vi "Code1Ps.vi"(11 "Code1 In":string) -> (1 "紙箱號碼":string, 2 "機種代號":string, 3 "機種名":string)   [LabVIEW 2014]
panel:
  out "Array":string[](array[string])
  out "appended array":bool[](array[boolean])
  out "array":string[](array[string])
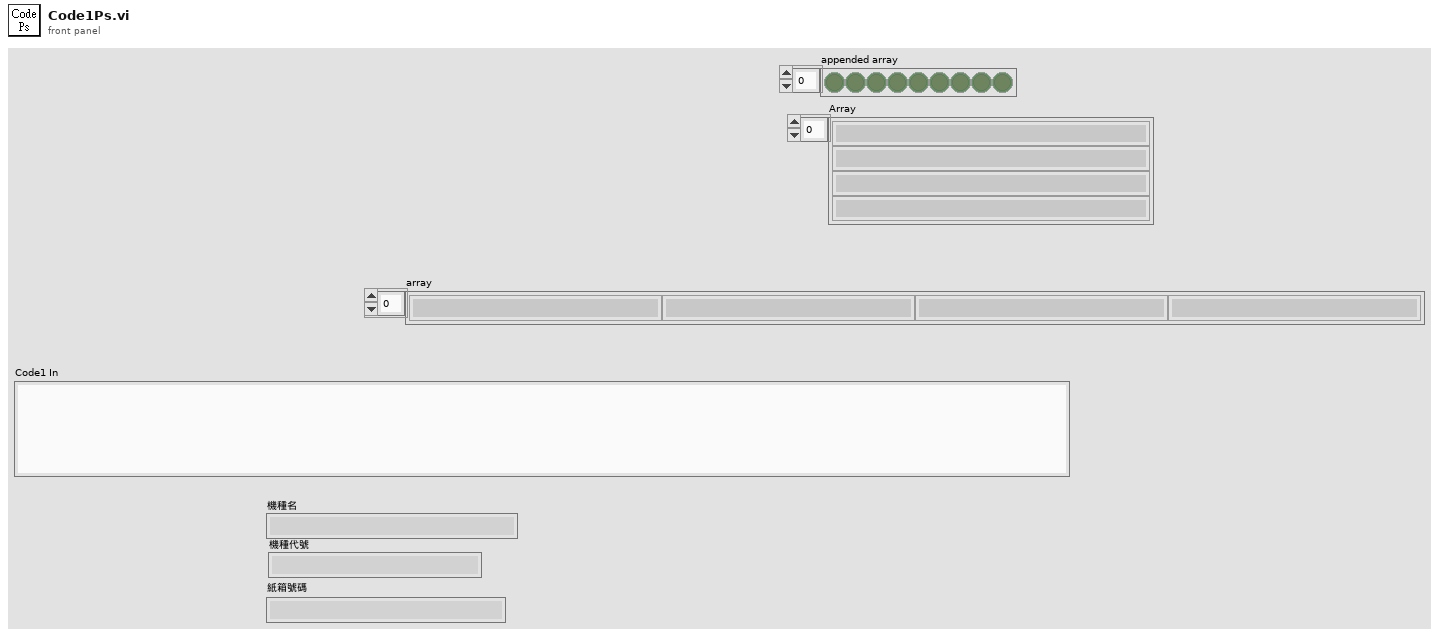
[diagram p1: front panel]
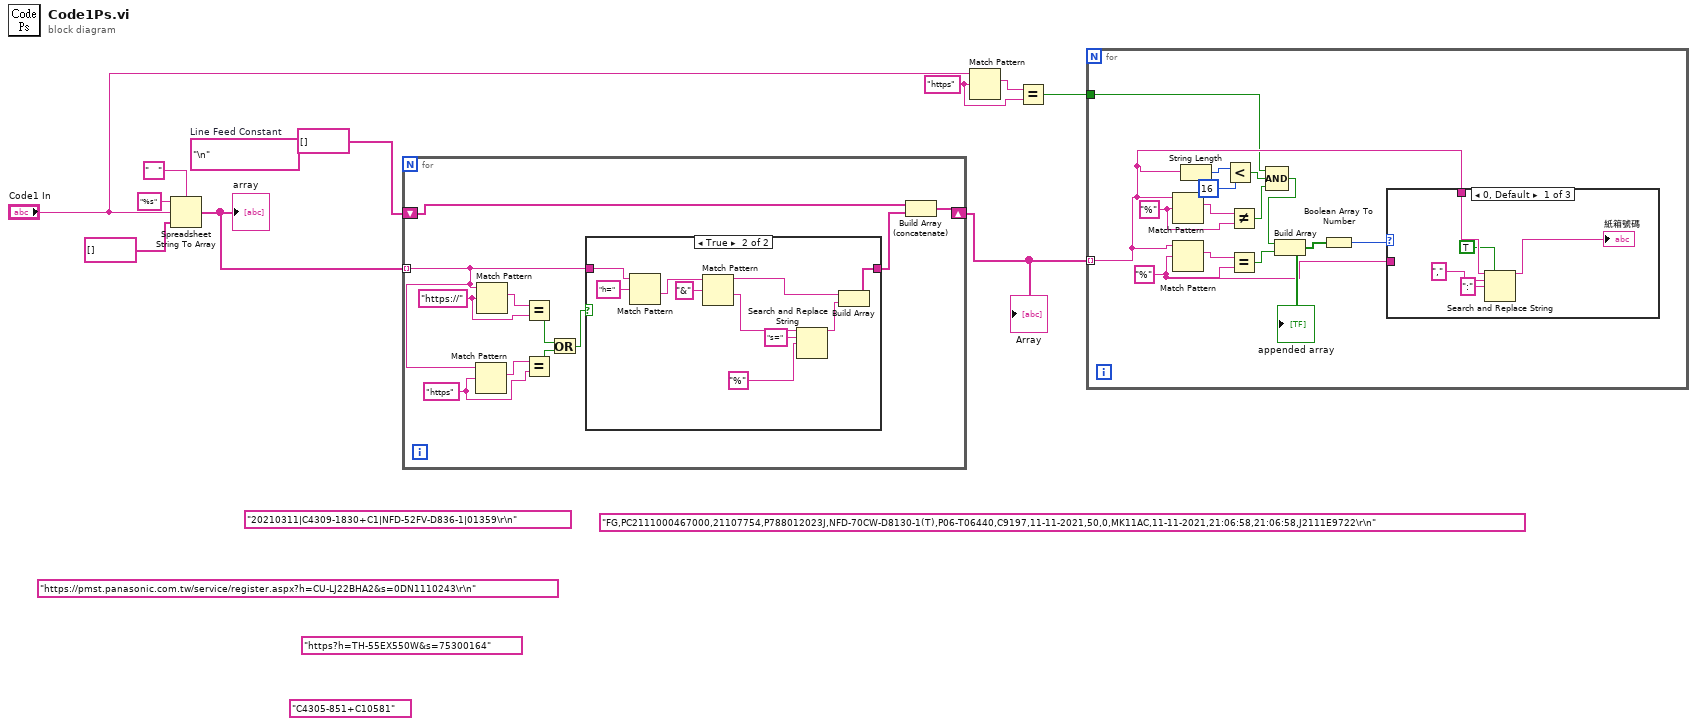
[diagram p0: block diagram]
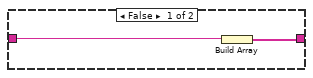
[diagram p2: hidden frame]
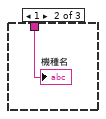
[diagram p3: hidden frame]
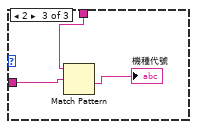
[diagram p4: hidden frame]
diagram:
  (unwired) "\n"  # Line Feed Constant
  (unwired) "FG,PC2111000467000,21107754,P788012023J,NFD-70CW-D8130-1(T),P06-T06440,C9197,11-11-2021,50,0,MK11AC,11-11-2021,21:06:58,21:06:58,J2111E9722\r\n" ("Code1 In")
  w3 = "https" ("regular expression")
  (unwired) "C4305-851+C10581"
  (unwired) "20210311|C4309-1830+C1|NFD-52FV-D836-1|01359\r\n" ("Code1 In")
  (unwired) "https://pmst.panasonic.com.tw/service/register.aspx?h=CU-LJ22BHA2&s=0DN1110243\r\n" ("Code1 In")
  (unwired) "https?h=TH-55EX550W&s=75300164" ("string")
  n1 = Spreadsheet String To Array(delimiter (Tab)="   ", format string="%s", spreadsheet string="Code1 In", array type (2D Dbl)=string[] []) -> (array=w8:string[])
  "array" <- w8
  n2 = for {
    tunnel: w8 -> [w16] mode=indexing
    shift-right: [w19] -> w6
    shift-left: string[] [] -> [w17]
    w14 = "https" ("regular expression")
    w21 = "https://" ("regular expression")
    n3 = Match Pattern(string=w16, regular expression=w14) -> (match substring=w15:string)  [unwired: 1 in, 3 out]
    n4 = Match Pattern(string=w16, regular expression=w21) -> (match substring=w20:string)  [unwired: 1 in, 3 out]
    n5 = Equal?(x=w20, y=w21) -> (x = y?=w13:bool)
    n6 = Equal?(x=w15, y=w14) -> (x = y?=w12:bool)
    n7 = Or(x=w13, y=w12) -> (x .or. y?=w11:bool)
    n8 = case shown="True" w11 {
      tunnel: [w22 w25] -> w18
      tunnel: w16 -> [w23 w24]
      frame False {
        n9 = Build Array(w23) -> (w22:string[])
      }
      frame True {
        n10 = Match Pattern(string=w24, regular expression="h=") -> (after substring=w27:string)  [unwired: 1 in, 3 out]
        n11 = Match Pattern(string=w27, regular expression="&") -> (before substring=w29:string, after substring=w30:string)  [unwired: 1 in, 2 out]
        n12 = Search and Replace String(input string=w30, search string="s=", replace string="%" ("replace string (\"\")")) -> (result string=w33:string)  [unwired: 5 in, 3 out]
        n13 = Build Array(w29, w33) -> (w25:string[])
      }
    }
    n14 = Build Array (concatenate)(w17, w18) -> (w19:string[])
  }
  "Array" <- w6
  n15 = Match Pattern(string="Code1 In", regular expression=w3) -> (match substring=w4:string)  [unwired: 1 in, 3 out]
  n16 = Equal?(x=w4, y=w3) -> (x = y?=w2:bool)
  n17 = for {
    tunnel: w6 -> [w41] mode=indexing
    tunnel: w2 -> [w35]
    w38 = "%" ("regular expression")
    w46 = "%" ("regular expression")
    n18 = Match Pattern(string=w41, regular expression=w46) -> (match substring=w47:string)  [unwired: 1 in, 3 out]
    n19 = Match Pattern(string=w41, regular expression=w38) -> (match substring=w45:string)  [unwired: 1 in, 3 out]
    n20 = String Length(string=w41) -> (length=w40:i32)
    n21 = Less?(x=w40, y=16) -> (x < y?=w36:bool)
    n22 = Not Equal?(x=w47, y=w46) -> (x != y?=w37:bool)
    n23 = Equal?(x=w45, y=w38) -> (x = y?=w44:bool)
    n24 = Compound Arithmetic op=AND(w35, w36, w37) -> (w34:bool)
    n25 = Build Array(w34, w44) -> (w43:bool[])
    "appended array" <- w43
    n26 = Boolean Array To Number(Boolean array=w43) -> (number=w42:u32)
    n27 = case shown="0, Default" w42 {
      tunnel: w41 -> [w52 w53 w56]
      tunnel: w38 -> [_ _ w55]
      frame 0, Default {
        n28 = Search and Replace String(replace all?=TRUE ("replace all? (F)"), input string=w52, search string=",", replace string=":" ("replace string (\"\")")) -> (result string=→"紙箱號碼":string)  [unwired: 4 in, 3 out]
      }
      frame 1 {
        "機種名" <- w53
      }
      frame 2 {
        n29 = Match Pattern(string=w56, regular expression=w55) -> (after substring=→"機種代號":string)  [unwired: 1 in, 3 out]
      }
    }
  }
